vi "sub_xydeg_to_gpsdeg.vi"(9 "dx - check":bool, 11 "xy deg in":dbl format="%.1f") -> (3 "gps deg out":dbl)   [LabVIEW 2019]
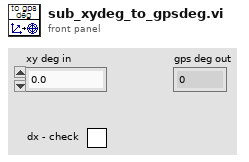
[diagram p1: front panel]
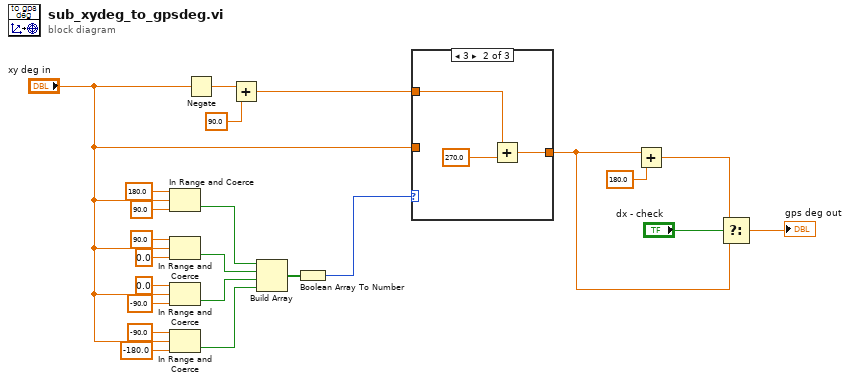
[diagram p0: block diagram]
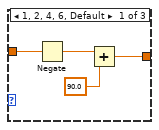
[diagram p2: hidden frame]
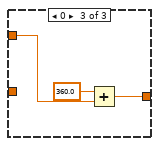
[diagram p3: hidden frame]
diagram:
  n1 = In Range and Coerce(upper limit=180.0, x="xy deg in", lower limit=90.0) -> (In Range?=w11:bool)  [unwired: 1 out]
  n2 = In Range and Coerce(upper limit=90.0, x="xy deg in", lower limit=0.0) -> (In Range?=w19:bool)  [unwired: 1 out]
  n3 = In Range and Coerce(upper limit=0.0, x="xy deg in", lower limit=-90.0) -> (In Range?=w16:bool)  [unwired: 1 out]
  n4 = In Range and Coerce(upper limit=-90.0, x="xy deg in", lower limit=-180.0) -> (In Range?=w6:bool)  [unwired: 1 out]
  n5 = Negate(x="xy deg in") -> (-x=w22:dbl)
  n6 = Add(x=w22, y=90.0) -> (x+y=w10:dbl)
  n7 = Build Array(w11, w19, w16, w6) -> (w15:bool[])
  n8 = Boolean Array To Number(Boolean array=w15) -> (number=w14:u32)
  n9 = case shown="3" w14 {
    tunnel: [w25 w29 w33] -> w2
    tunnel: "xy deg in" -> [w24 _ _]
    tunnel: w10 -> [_ w28 w31]
    frame 1, 2, 4, 6, Default {
      n10 = Negate(x=w24) -> (-x=w27:dbl)
      n11 = Add(x=w27, y=90.0) -> (x+y=w25:dbl)
    }
    frame 3 {
      n12 = Add(x=w28, y=270.0) -> (x+y=w29:dbl)
    }
    frame 0 {
      n13 = Add(x=360.0, y=w31) -> (x+y=w33:dbl)
    }
  }
  n14 = Add(x=w2, y=180.0) -> (x+y=w1:dbl)
  n15 = Select(t=w1, s="dx - check", f=w2) -> (s? t:f=→"gps deg out":dbl)
